vi "Append Numeric Table to Report.vi"(0 "report in":refnum<class "NI_Excel.lvclass">, 1 "column width (1)":dbl=1.0 format="%.2f", 2 "measurement system":u16(ring)=2 caption="measurement system for column width (Default)" items=["US", "Metric", "Default"], 3 "MS Office parameters":T2, 5 "column headers":string[](array[string]), 7 "row headers":string[](array[string]), 9 "numerical data":dbl[][](array[numeric]) format="%.2f", 11 "error in (no error)":errorcluster, 12 "format string (%.3f)":string="%.3f", 13 "separate page?":bool, 14 "show grid lines":bool=TRUE) -> (4 "report out":refnum<class "NI_Excel.lvclass">, 8 "range (wd) - start (xl)":T1, 10 "end (xl)":cluster{"row (xl) ":i32, "col (xl) ":i32}, 15 "error out":errorcluster)   [LabVIEW 2023, in "NI_Excel.lvclass"]
doc: "Appends a 2D array to a report as a table with the given column width. You can use this polymorphic VI to append an array of strings or numbers. The data type you wire to the <B>text data</B> input determines the polymorphic instance to use."
uses:
  NI_Excel.lvclass
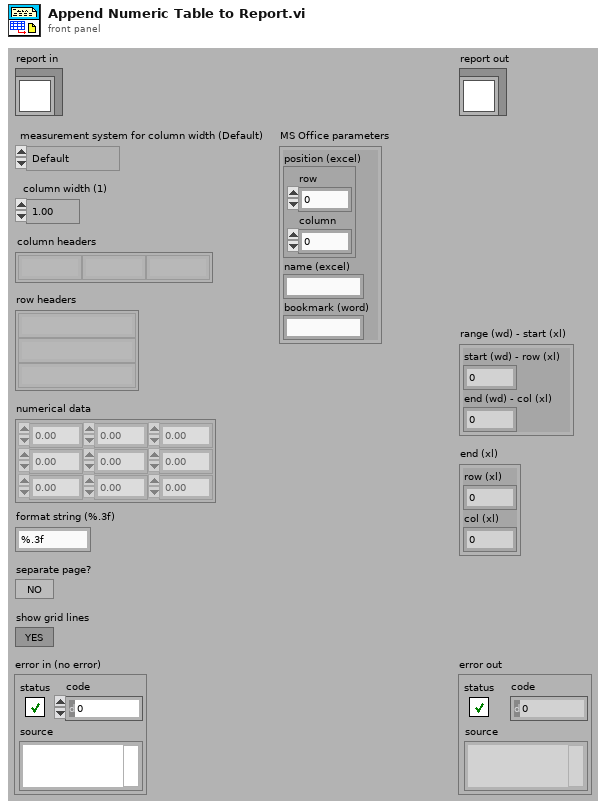
[diagram p1: front panel]
types:
  T1 = cluster{"start (wd) - row (xl) ":i32, "end (wd) - col (xl) ":i32}
  T2 = cluster{"position (excel)":cluster{"row":i32, "column":i32}, "name (excel)":string, "bookmark (word)":string}
  T3 = typedef "NI_ReportGenerationCore.lvlib/Report Data Members.ctl" = cluster{"font":T4, "from template?":bool}
  T4 = typedef "NI_ReportGenerationCore.lvlib/font.ctl" = cluster{"font name":string, "font size":dbl, "bold":u16, "italic":u16, "underline":u16, "strike through":u16, "font color":u32}
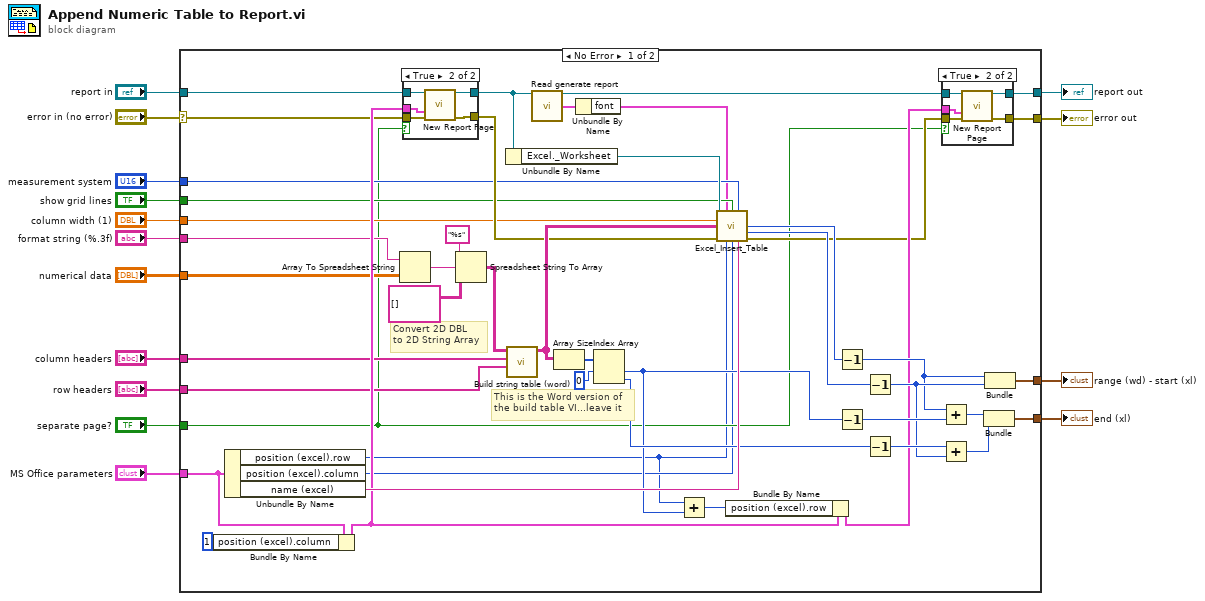
[diagram p0: block diagram]
diagram:
  n1 = case shown="No Error" "error in (no error)" {
    selector: "error in (no error)" -> [w38 w77]
    tunnel: [w37 w77] -> w14
    tunnel: [w22 w76] -> w12
    tunnel: "report in" -> [w36 w76]
    tunnel: "show grid lines" -> [w30 _]
    tunnel: "format string (%.3f)" -> [w26 _]
    tunnel: "row headers" -> [w29 _]
    tunnel: "column headers" -> [w28 _]
    tunnel: "numerical data" -> [w27 _]
    tunnel: "column width (1)" -> [w25 _]
    tunnel: "MS Office parameters" -> [w35 _]
    tunnel: [w32 _] -> w4
    tunnel: [w31 _] -> w3
    tunnel: "measurement system" -> [w24 _]
    tunnel: "separate page?" -> [w23 _]
    frame No Error {
      # "This is the Word version of\nthe build table VI...leave it"
      # "Convert 2D DBL\nto 2D String Array"
      n2 = Bundle By Name(cluster=w35, "position (excel).column"=1) -> (w39:T2)
      n3 = Unbundle By Name(w35) -> ("position (excel).row"=w20:i32, "position (excel).column"=w21:i32, "name (excel)"=w57:string)
      n4 = Array To Spreadsheet String(array=w27, 3:w26) -> (spreadsheet string=w53:string)  [unwired: 1 out]
      n5 = case shown="True" w23 {
        tunnel: w36 -> [w70 w75]
        tunnel: w38 -> [w69 w74]
        tunnel: [w70 w73] -> w19
        tunnel: [w69 w72] -> w33
        tunnel: w39 -> [_ w71]
        frame False {
        }
        frame True {
          n6 = call-dynamic "New Report Page.vi"("report in"=w75, "MS Office parameters"=w71, "error in (no error)"=w74) -> ("report out"=w73:refnum<class "NI_Excel.lvclass">, "error out"=w72:errorcluster)  [unwired: 11 in]
        }
      }
      n7 = Spreadsheet String To Array(format string="%s", spreadsheet string=w53, array type (2D Dbl)=string[][] [] ("output table")) -> (array=w54:string[][])  [unwired: 1 out]
      n8 = Unbundle By Name(w19) -> ("Excel._Worksheet"=w59:refnum<k7>)
      n9 = call <vilib>:"Build string table (word).vi"("row headers"=w29, "column headers"=w28, "text data"=w54) -> ("output table"=w58:string[][])  [unwired: 1 in, 7 out]
      n10 = call-dynamic "Read generate report.vi"("report in"=w19) -> ("report out"=w18:refnum<class "NI_Excel.lvclass">, "generate report"=w17:T3)  [unwired: 12 in, 1 out]
      n11 = Array Size(array=w58) -> (size(s)=w43:i32[])
      n12 = Unbundle By Name(w17) -> ("font"=w16:T4)
      n13 = Index Array(array=w43, index #1=0 ("Index")) -> (element #1=w51:i32, element #2=w52:i32)  [unwired: 1 in]
      n14 = Add(x=w20, y=w51) -> (x+y=w41:i32)
      n15 = call <vilib>:"Excel_Insert_Table.vi"("worksheet"=w59, "font"=w16, "show grid lines"=w30, "measurement system"=w24, "column width (1)"=w25, "table"=w58, "error in (no error)"=w33, "Start row"=w20, "Start column"=w21, "name"=w57) -> ("Row"=w60:i32, "Column"=w61:i32, "error out"=w34:errorcluster)  [unwired: 3 out]
      n16 = Bundle By Name(cluster=w39, "position (excel).row"=w41) -> (w42:T2)
      n17 = Decrement(x=w60) -> (x-1=w47:i32)
      n18 = Decrement(x=w51) -> (x-1=w49:i32)
      n19 = Decrement(x=w61) -> (x-1=w48:i32)
      n20 = Decrement(x=w52) -> (x-1=w50:i32)
      n21 = Add(x=w47, y=w49) -> (x+y=w45:i32)
      n22 = Add(x=w50, y=w48) -> (x+y=w46:i32)
      n23 = case shown="True" w23 {
        tunnel: [w63 w68] -> w22
        tunnel: [w62 w67] -> w37
        tunnel: w34 -> [w62 w66]
        tunnel: w18 -> [w63 w65]
        tunnel: w42 -> [_ w64]
        frame False {
        }
        frame True {
          n24 = call-dynamic "New Report Page.vi"("report in"=w65, "MS Office parameters"=w64, "error in (no error)"=w66) -> ("report out"=w68:refnum<class "NI_Excel.lvclass">, "error out"=w67:errorcluster)  [unwired: 11 in]
        }
      }
      n25 = Bundle(w45, w46) -> (w31:cluster{i32, i32})  [unwired: 1 out]
      n26 = Bundle(w47, w48) -> (w32:cluster{i32, i32})  [unwired: 1 out]
    }
    frame Error {
    }
  }
  "error out" <- w14
  "report out" <- w12
  "end (xl)" <- w3
  "range (wd) - start (xl)" <- w4
